vi "Value to timestamp.vi"(1 "TimeStamp":dbl) -> (0 "Time Stamp":timestamp)   [LabVIEW 2020]
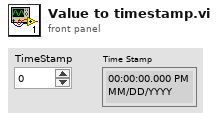
[diagram p1: front panel]
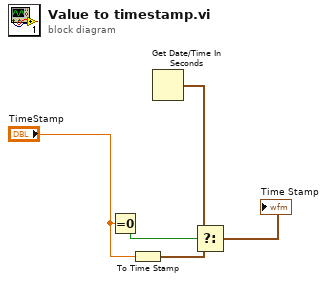
[diagram p0: block diagram]
diagram:
  n1 = Equal To 0?(x="TimeStamp") -> (x = 0?=w4:bool)
  n2 = To Time Stamp(1:"TimeStamp") -> (0:w3:timestamp)
  n3 = Get Date/Time In Seconds() -> (seconds since 1Jan1904=w1:timestamp)
  n4 = Select(t=w1, s=w4, f=w3) -> (s? t:f=→"Time Stamp":timestamp)
